vi "cb_SPIEnginewithDIO.vi"() -> ()   [LabVIEW 2013]
uses:
  <vilib>/Platform/TimedLoop/XDataNode/XDataNode.xnode
  <vilib>/Platform/TimedLoop/XDataNode/nitl_modes.ctl
  <vilib>/Platform/TimedLoop/XDataNode/XDNodeRunTimeDep.lvlib
  <vilib>/Platform/TimedLoop/XDataNode/wakeup.ctl
  <vilib>/Platform/TimedLoop/XDataNode/timing_clust.ctl
  DIO/SPI Digital IO Lines.ctl
  DIO/SPI DIO Enable Lines.ctl
  Program Files (x86)/National Instruments/LabVIEW 2014/user.lib/_NI SPI IP/FPGA/Controllers/Public/Spi Master Outputs.ctl
  Program Files (x86)/National Instruments/LabVIEW 2014/user.lib/_NI SPI IP/FPGA/Controllers/NI SPI IP (FPGA).lvlib
  Program Files (x86)/National Instruments/LabVIEW 2014/user.lib/_NI SPI IP/FPGA/Controllers/Public/Transfer Settings.ctl
panel:
  out "Read Data":u64
  out "Read Data Valid?":bool
  in  "start":bool=TRUE
  out "IP Strobe Count":u64
  out "NumRq":u64
  in  "SPI PHY Settings":T1={"Divide Value"=20, "Transfer Length (bits)"=32, "CS Asserted Polarity"=TRUE, "Clock Polarity (CPOL)"=TRUE, "Clock Phase (CPHA)"=FALSE, "Lengthen MISO Setup"=FALSE, "Direction Change Bit"=0, "MOSI Starts as Output"=FALSE, "Tristatable MOSI"=FALSE} {"Direction Change Bit" max=64 step=1; "Transfer Length (bits)" min=1 max=64 step=1}
  in  "stop":bool
  out "spi output":T2
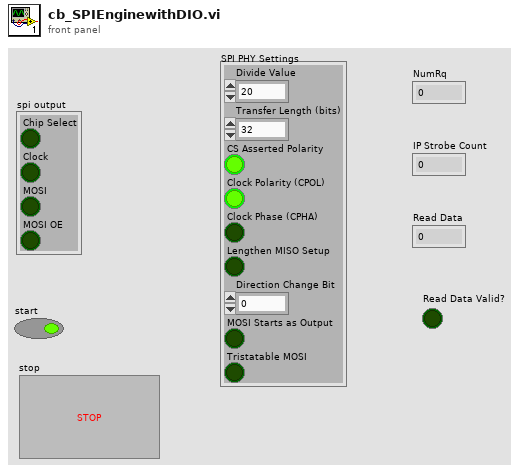
[diagram p1: front panel]
types:
  T1 = typedef "NI SPI IP (FPGA).lvlib/Transfer Settings.ctl" = cluster{"Divide Value":u8, "Transfer Length (bits)":u8, "CS Asserted Polarity":bool, "Clock Polarity (CPOL)":bool, "Clock Phase (CPHA)":bool, "Lengthen MISO Setup":bool, "Direction Change Bit":u8, "MOSI Starts as Output":bool, "Tristatable MOSI":bool}
  T2 = typedef "NI SPI IP (FPGA).lvlib/Spi Master Outputs.ctl" = cluster{"Chip Select":bool, "Clock":bool, "MOSI":bool, "MOSI OE":bool}
  T3 = typedef "SPI DIO Enable Lines.ctl" = cluster{"SCLK_en":refnum<k21>, "MISO_en":refnum<k21>, "MOSI_en":refnum<k21>, "CS0_en":refnum<k21>, "CS1_en":refnum<k21>, "CS2_en":refnum<k21>, "CS3_en":refnum<k21>, "CS4_en":refnum<k21>, "CS5_en":refnum<k21>}
  T4 = typedef "SPI Digital IO Lines.ctl" = cluster{"SCLK":refnum<k21>, "MISO":refnum<k21>, "MOSI":refnum<k21>, "CS 0":refnum<k21>, "CS 1":refnum<k21>, "CS 2":refnum<k21>, "CS 3":refnum<k21>, "CS 4":refnum<k21>, "CS 5":refnum<k21>}
  T5 = typedef "XDNodeRunTimeDep.lvlib/timing_clust.ctl" = cluster{"Expected End [f-1]":u64, "Actual End [f-1]":u64, "Finished Late? [f-1]":bool, "Expected End [i-1]":u64, "Actual End [i-1]":u64, "Finished Late? [i-1]":bool, "Expected Start [i]":u64, "Actual Start [i]":u64, "Expected Start [f]":u64, "Actual Start [f]":u64, "Source Name":string, "Structure Name":string, "Period":i64, "Deadline":i64, "Offset":i64, "Start":i64, "Priority":i32, "Timeout":i32, "Mode":T6, "Wakeup Reason":T7, "Error":errorcluster, "Source Type":string, "Secondary Source Type":string, "Global End Time":u64, "Global Start Time":u64, "Frame Duration":u64, "Iteration Duration":u64, "Assigned CPU":i32, "I/O Scan Engine Mode":u32}
  T6 = typedef "XDNodeRunTimeDep.lvlib/nitl_modes.ctl" = enum32{"No Change", "Process missed periods, maintain original phase", "Discard missed periods, maintain original phase", "Process missed periods, ignore original phase", "Discard missed periods, ignore original phase"}
  T7 = typedef "XDNodeRunTimeDep.lvlib/wakeup.ctl" = enum32{"Normal", "Aborted", "Asynchronous wakeup", "Timing source error", "Timed loop error", "Timeout"}
  T8 = typedef "Internal Data (SPI API).ctl" = cluster{"DLU To SPI Engine Data FIFO":refnum<k21>, "SPI Engine to DLU Data FIFO":refnum<k21>, "Data to SPI Engine (Cache) Register":refnum<k21>, "SPI PHY Settings to SPI Engine (Cahche) Register":refnum<k21>}
  T9 = typedef "NI SPI IP (FPGA).lvlib/Spi Master Inputs.ctl" = cluster{"MISO":bool}
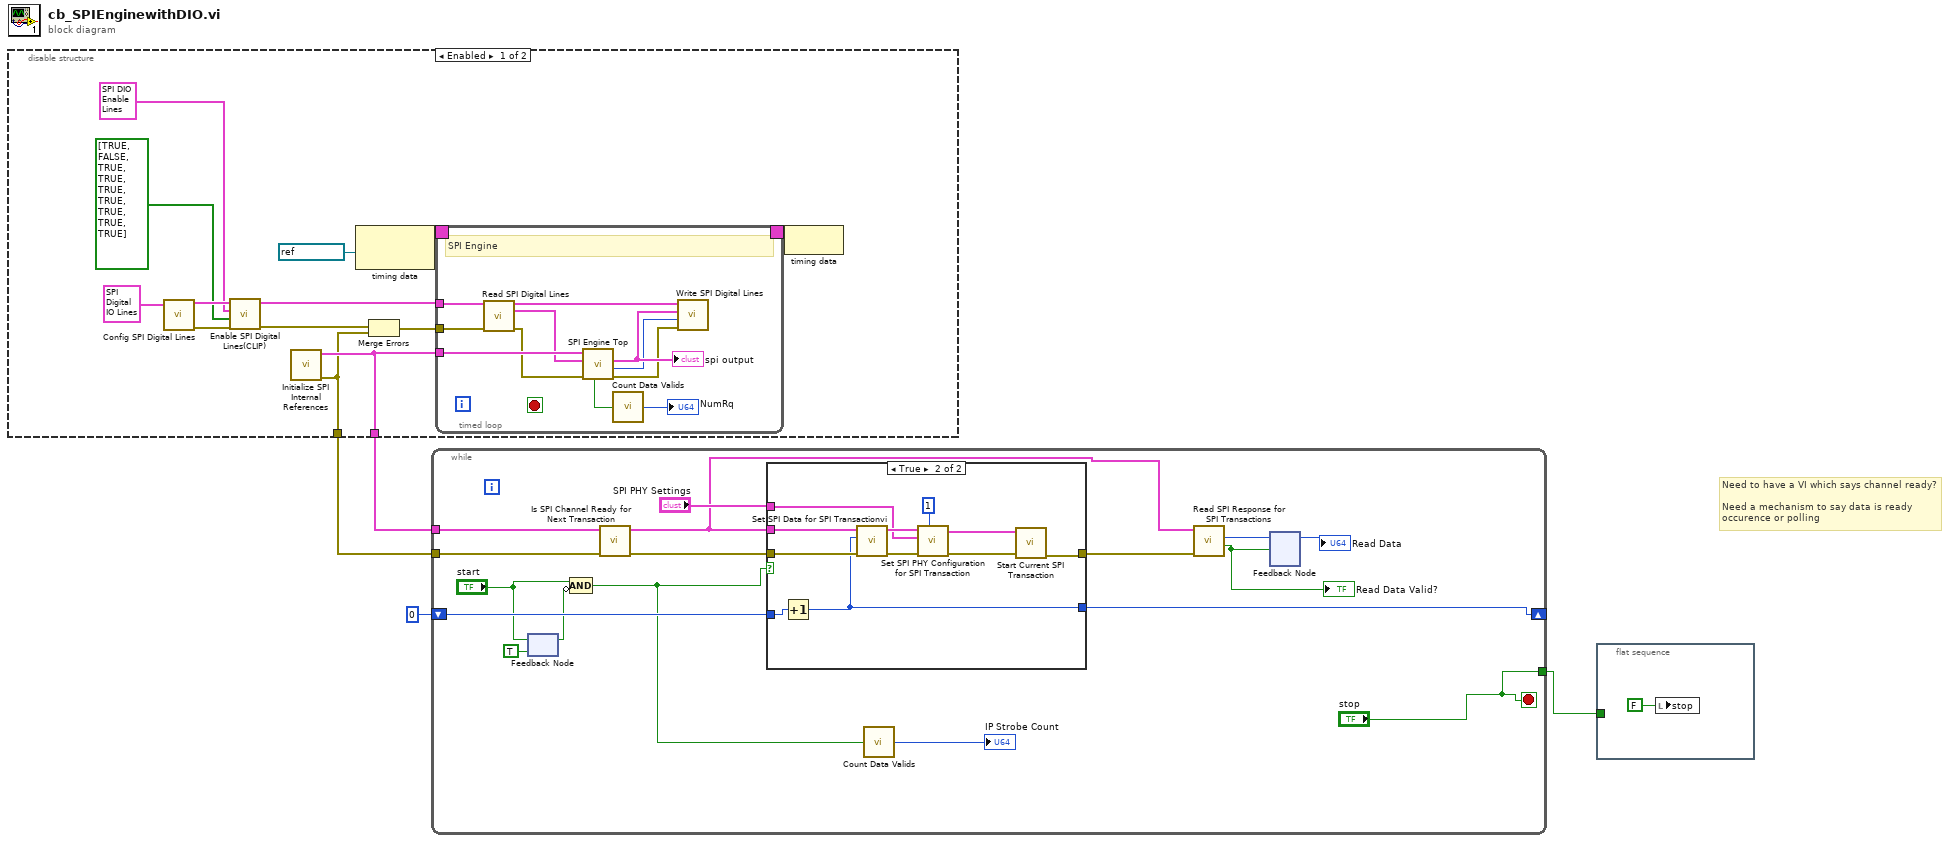
[diagram p0: block diagram]
diagram:
  # "Need to have a VI which says channel ready?\n\nNeed a mechanism to say data is ready\noccurence or polling"
  n1 = disable-structure shown="Enabled" {
    disable-tunnel: [w15 _] -> w4
    disable-tunnel: [w14 _] -> w1
    frame Enabled {
      n2 = call "Config SPI Digital Lines.vi"("SPI DIO Lines"=T4 {"SCLK"="sbRIO-9651 Socket\\PMOD1_Pin1_out", "MISO"="sbRIO-9651 Socket\\PMOD1_Pin2_in", "MOSI"="sbRIO-9651 Socket\\PMOD1_Pin3_out", "CS 0"="sbRIO-9651 Socket\\PMOD1_Pin4_out", "CS 1"="sbRIO-9651 Socket\\PMOD1_Pin4_out", "CS 2"="sbRIO-9651 Socket\\PMOD1_Pin4_out", "CS 3"="sbRIO-9651 Socket\\PMOD1_Pin4_out", "CS 4"="sbRIO-9651 Socket\\PMOD1_Pin4_out", "CS 5"="sbRIO-9651 Socket\\PMOD1_Pin4_out"} ("Chip Select DIO Lines")) -> ("error out"=w9:errorcluster, "Chip Select DIO Lines"=w10:T4)  [unwired: 9 in]
      n3 = call "Enable SPI Digital Lines(CLIP).vi"("error in"=w9, "Enable"=bool[] [TRUE, FALSE, TRUE, TRUE, TRUE, TRUE, TRUE, TRUE, TRUE], "Enable Lines"=T3 {"SCLK_en"="sbRIO-9651 Socket\\PMOD1_Pin1_enable", "MISO_en"="sbRIO-9651 Socket\\PMOD1_Pin2_enable", "MOSI_en"="sbRIO-9651 Socket\\PMOD1_Pin3_enable", "CS0_en"="sbRIO-9651 Socket\\PMOD1_Pin4_enable", "CS1_en"="sbRIO-9651 Socket\\PMOD1_Pin4_enable", "CS2_en"="sbRIO-9651 Socket\\PMOD1_Pin4_enable", "CS3_en"="sbRIO-9651 Socket\\PMOD1_Pin4_enable", "CS4_en"="sbRIO-9651 Socket\\PMOD1_Pin4_enable", "CS5_en"="sbRIO-9651 Socket\\PMOD1_Pin4_enable"}, "SPI DIO Lines"=w10) -> ("error out"=w6:errorcluster, "Chip Select DIO Lines"=w7:T4)  [unwired: 6 in]
      n4 = call "Initialize SPI Internal References.vi"() -> ("error out"=w14:errorcluster, "SPI API References"=w15:T8)  [unwired: 10 in]
      n5 = node-c288(refnum<k21> "120MHz" ("Source Name")) -> (w17:T5)
      n6 = Merge Errors(w6, w14) -> (w13:errorcluster)
      n7 = timed-loop {
        tunnel: w15 -> [w24]
        tunnel: w13 -> [w22]
        tunnel: w7 -> [w26]
        timing: w17 -> [_]
        timing-out: [_] -> w16
        stop <- _ stop-if-true
        # "SPI Engine"
        n8 = call "Read SPI Digital Lines.vi"("Chip Select DIO Lines"=w26, "error in"=w22) -> ("Chip Select DIO Lines Out"=w27:T4, "SPI Read Data"=w23:T9, "error out"=w21:errorcluster)  [unwired: 11 in]
        n9 = call "SPI Engine Top.vi"("error in"=w21, "SPI Read Data"=w23, "SPI API References"=w24) -> ("error out"=w20:errorcluster, "Chip Select ID"=w18:u8, "SPI DIO Output"=w25:T2, "New Input Data Received?"=w19:bool)  [unwired: 3 in, 2 out]
        "spi output" <- w25
        n10 = call "Count Data Valids.vi"("Data Valid"=w19) -> ("Counter"=→"NumRq":u64)  [unwired: 14 in]
        n11 = call "Write SPI Digital Lines.vi"("error in"=w20, "CS Index"=w18, "spi output"=w25, "Chip Select DIO Lines"=w27) -> ()  [unwired: 6 in, 2 out]
      }
      n12 = node-c288(w16) -> ()
    }
    frame Disabled {
    }
  }
  n13 = while {
    tunnel: w4 -> [w49]
    tunnel: ["stop"] -> w3
    tunnel: w1 -> [w48]
    shift-right: [w45] -> _
    shift-left: u8 0 -> [w46]
    stop <- "stop" stop-if-true
    n14 = feedback-in #1("start") -> ()
    n15 = feedback #1(TRUE ("start")) -> (w42:bool)
    n16 = Compound Arithmetic op=AND("start", invert w42) -> (w40:bool)
    n17 = call "Is SPI Channel Ready for Next Transaction.vi"("error in"=w48, "Private Data In"=w49) -> ("error out"=w47:errorcluster, "Private Data Out"=w36:T8)  [unwired: 6 in, 2 out]
    n18 = case shown="True" w40 {
      tunnel: w36 -> [_ w63]
      tunnel: "SPI PHY Settings" -> [_ w60]
      tunnel: [_ w55] -> w44
      tunnel: w47 -> [_ w58]
      tunnel: w46 -> [w52 w57]
      tunnel: [w52 w56] -> w45
      frame False {
      }
      frame True {
        n19 = Increment(x=w57) -> (x+1=w56:u8)
        n20 = call "Set SPI Data for SPI Transactionvi.vi"("error in"=w58, "Data In"=w56, "Private Data In"=w63) -> ("error out"=w61:errorcluster, "Private Data Out"=w62:T8)  [unwired: 7 in]
        n21 = call "Set SPI PHY Configuration for SPI Transaction.vi"("Chip Select"=u8 1, "error in"=w61, "SPI PHY Settings"=w60, "Private Data In"=w62) -> ("error out"=w53:errorcluster, "Private Data Out"=w54:T8)  [unwired: 6 in]
        n22 = call "Start Current SPI Transaction.vi"("error in"=w53, "Private Data In"=w54) -> ("error out"=w55:errorcluster)  [unwired: 7 in, 2 out]
      }
    }
    n23 = call "Count Data Valids.vi"("Data Valid"=w40) -> ("Counter"=→"IP Strobe Count":u64)  [unwired: 14 in]
    n24 = call "Read SPI Response for SPI Transactions.vi"("error in"=w44, "Private Data In"=w36) -> ("Read Data Valid?"=w39:bool, "Read Data"=w38:u64)  [unwired: 6 in, 2 out]
    "Read Data Valid?" <- w39
    n25 = feedback-in #2(w38, w39) -> ()
    n26 = feedback #2() -> (→"Read Data":u64)  [unwired: 1 in]
  }
  n27 = flat-sequence {
    tunnel: w3 -> [_]
    frame #0 {
      n28 = local write "stop"(FALSE ("stop")) -> ()
    }
  }
